vi "Profile Table Interpolation.vi"(7 "Profile Select":dbl, 8 "Error In":errorcluster, 10 "x":dbl, 11 "Profiles []":cluster{"Profile":dbl[][]}[](array[cluster])) -> (0 "Error Out":errorcluster, 1 "Interpolated y-MaxLimit":dbl, 2 "Interpolated y-MinLimit":dbl, 3 "Interpolated y":dbl)   [LabVIEW 2019, in "Profile Interpolation Engine.lvlib"]
doc: "This VI takes a set of Profiles and uses those to interpolate appropriate y, y-MaxLimit, y-MinLimit from a given x value."
uses:
  Profile Interpolation Engine.lvlib
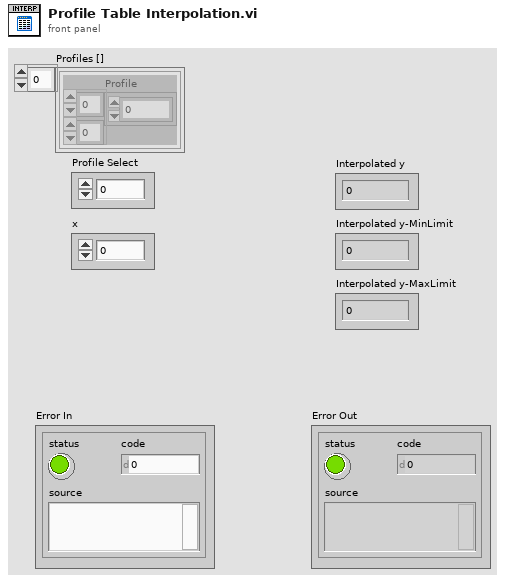
[diagram p1: front panel]
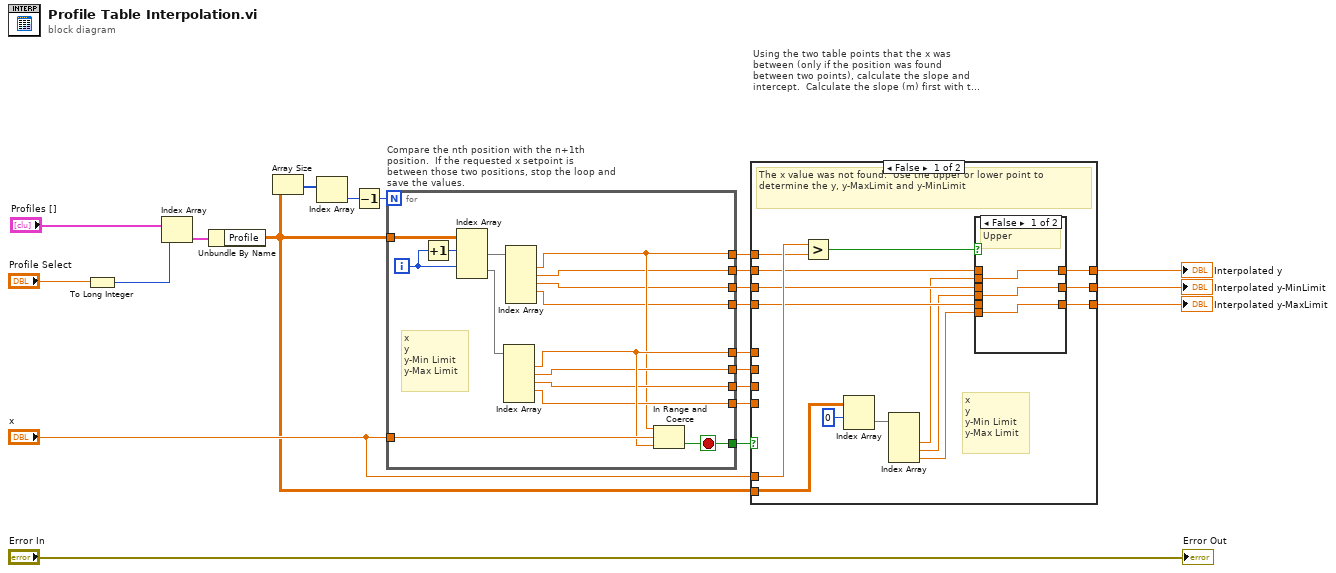
[diagram p0: block diagram]
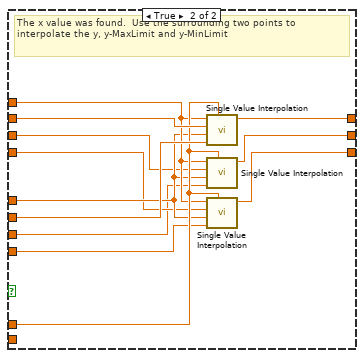
[diagram p3: hidden frame]
diagram:
  n1 = To Long Integer(number="Profile Select") -> (32bit integer=w7:i32)
  n2 = Index Array(array="Profiles []", index=w7) -> (element=w6:cluster{"Profile":dbl[][]})
  n3 = Unbundle By Name(w6) -> ("Profile"=w2:dbl[][])
  n4 = Array Size(array=w2) -> (size(s)=w5:i32[])
  n5 = Index Array(array=w5) -> (element=w4:i32)  [unwired: 1 in]
  n6 = Decrement(x=w4) -> (x-1=w3:i32)
  n7 = for "Compare the nth position with the n+1th position.  If the requested x setpoint is between those two positions, stop the loop and save the values." {
    N: w3 -> [_]
    tunnel: "x" -> [w37]
    tunnel: [w26] -> w19
    tunnel: [w25] -> w20
    tunnel: [w30] -> w21
    tunnel: [w29] -> w22
    tunnel: [w36] -> w15
    tunnel: [w24] -> w14
    tunnel: [w23] -> w13
    tunnel: [w28] -> w12
    tunnel: [w27] -> w11
    tunnel: w2 -> [w35]
    i -> [w33]
    stop <- w36 stop-if-true
    # "x\ny\ny-Min Limit\ny-Max Limit"
    n8 = Increment(x=w33) -> (x+1=w34:i32)
    n9 = Index Array(array=w35, index (row) #1=w34, index (row) #2=w33) -> (element #1=w32:dbl[], element #2=w31:dbl[])  [unwired: 2 in]
    n10 = Index Array(array=w31) -> (element #1=w30:dbl, element #2=w29:dbl, element #3=w28:dbl, element #4=w27:dbl)  [unwired: 5 in, 1 out]
    n11 = Index Array(array=w32) -> (element #1=w26:dbl, element #2=w25:dbl, element #3=w24:dbl, element #4=w23:dbl)  [unwired: 5 in, 1 out]
    n12 = In Range and Coerce(upper limit=w26, x=w37, lower limit=w30) -> (In Range?=w36:bool)  [unwired: 1 out]
  }
  n13 = case "Using the two table points that the x was between (only if the position was found between two points), calculate the slope and intercept.  Calculate the slope (m) first with the formula (y2-y1)/(x2-x1).  Use the slope and the upper of the two table points to calculate the intercept (b).  Once m and b are calculated, use the formula y=mx+b with the original (x) to calculate the interpolated (y).\n\nIf the position wasn't found between two points, use the load  from whichever end point it was closest to." shown="False" w15 {
    tunnel: w22 -> [_ w68]
    tunnel: w21 -> [_ w63]
    tunnel: w20 -> [w48 w70]
    tunnel: w19 -> [w50 w64]
    tunnel: "x" -> [w52 w67]
    tunnel: [w49 w69] -> w17
    tunnel: w14 -> [w47 w62]
    tunnel: w13 -> [w46 w61]
    tunnel: w12 -> [_ w60]
    tunnel: w11 -> [_ w59]
    tunnel: [w45 w66] -> w9
    tunnel: [w44 w65] -> w10
    tunnel: w2 -> [w43 _]
    frame False {
      # "x\ny\ny-Min Limit\ny-Max Limit"
      # "The x value was not found.  Use the upper or lower point to determine the y, y-MaxLimit and y-MinLimit"
      n14 = Greater?(x=w52, y=w50) -> (0:w51:bool)
      n15 = Index Array(array=w43, index (row)=0) -> (element=w41:dbl[])  [unwired: 1 in]
      n16 = Index Array(array=w41) -> (element #2=w40:dbl, element #3=w39:dbl, element #4=w38:dbl)  [unwired: 4 in, 1 out]
      n17 = case shown="False" w51 {
        tunnel: [w55 w58] -> w49
        tunnel: w48 -> [_ w58]
        tunnel: w40 -> [w55 _]
        tunnel: w47 -> [_ w57]
        tunnel: w46 -> [_ w56]
        tunnel: w39 -> [w53 _]
        tunnel: w38 -> [w54 _]
        tunnel: [w53 w57] -> w45
        tunnel: [w54 w56] -> w44
        frame False {
          # "Upper"
        }
        frame True {
          # "Upper"
        }
      }
    }
    frame True {
      # "The x value was found.  Use the surrounding two points to interpolate the y, y-MaxLimit and y-MinLimit"
      n18 = call "Single Value Interpolation.vi"("x"=w67, "Lower Value"=w68, "Lower Position"=w63, "Upper Value"=w70, "Upper Position"=w64) -> ("Interpolated Value"=w69:dbl)  [unwired: 6 in]
      n19 = call "Single Value Interpolation.vi"("x"=w67, "Lower Value"=w60, "Lower Position"=w63, "Upper Value"=w62, "Upper Position"=w64) -> ("Interpolated Value"=w66:dbl)  [unwired: 6 in]
      n20 = call "Single Value Interpolation.vi"("x"=w67, "Lower Value"=w59, "Lower Position"=w63, "Upper Value"=w61, "Upper Position"=w64) -> ("Interpolated Value"=w65:dbl)  [unwired: 6 in]
    }
  }
  "Interpolated y" <- w17
  "Interpolated y-MinLimit" <- w9
  "Interpolated y-MaxLimit" <- w10
  "Error Out" <- "Error In"
